vi "Get Format Test Settings.vi"(8 "Error In":errorcluster, 11 "Data Channel Ref In":T1 format="%.0x") -> (0 "Error Out":errorcluster, 2 "Data Channel Settings":T2, 3 "Data Channel Ref Out":T1 format="%.0x")   [LabVIEW 2018, in "Instrument Addon Scripting API Channels Unit Tests.lvclass"]
uses:
  Instrument Addon Scripting API Channels Unit Tests.lvclass
  <vilib>/NI Veristand/Custom Device API/Custom Device Item Ref.ctl
  APIs/Scripting API/TypeDefs/Array Format Settings.ctl
  APIs/Scripting API/TypeDefs/Array Element.ctl
  <vilib>/NI Veristand/Custom Device API/Get Item Property (String).vi
  <vilib>/NI Veristand/Custom Device API/Custom Device API.lvlib
  APIs/Scripting API/Instrument Addon Scripting API.lvlib
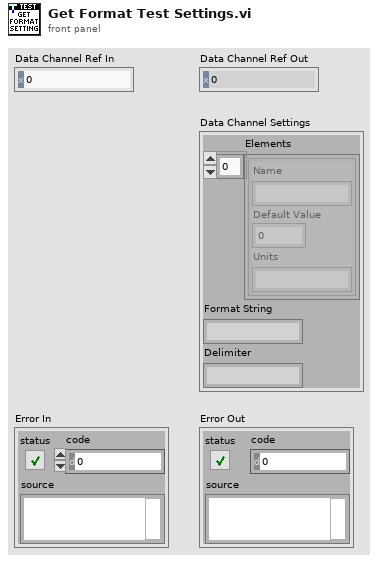
[diagram p1: front panel]
types:
  T1 = typedef "Custom Device API.lvlib/Custom Device Item Ref.ctl" = u64
  T2 = typedef "Instrument Addon Scripting API.lvlib/Array Format Settings.ctl" = cluster{"Elements":T3[], "Format String":string, "Delimiter":string}
  T3 = typedef "Instrument Addon Scripting API.lvlib/Array Element.ctl" = cluster{"Name":string, "Default Value":dbl, "Units":string}
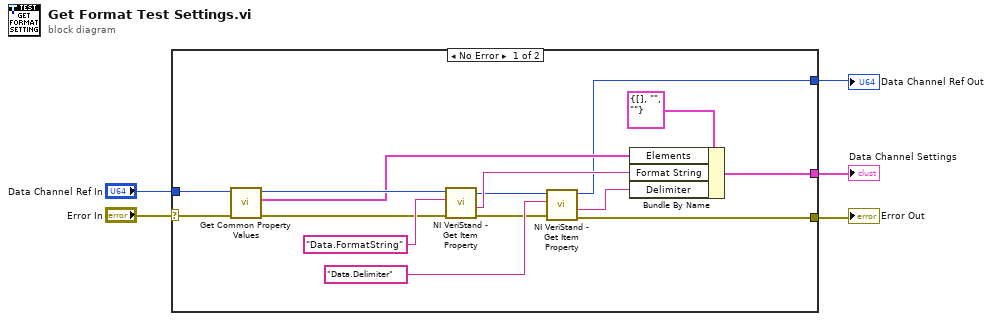
[diagram p0: block diagram]
diagram:
  n1 = case shown="No Error" "Error In" {
    selector: "Error In" -> [w6 w21]
    tunnel: [w20 _] -> w5
    tunnel: [w17 w21] -> w4
    tunnel: "Data Channel Ref In" -> [w11 w22]
    tunnel: [w7 w22] -> w1
    frame No Error {
      n2 = call "Get Common Property Values.vi"("Error In"=w6, "Data Channel  Ref in"=w11) -> ("error out"=w10:errorcluster, "Array Out"=w8:T3[], "Data Channel Ref Out"=w9:u64)  [unwired: 7 in]
      n3 = call-poly <vilib>:"NI VeriStand - Get Item Property.vi"("error in (no error)"=w10, "Property Name"="Data.FormatString", "Item Ref in"=w9) -> ("error out"=w13:errorcluster, "Value"=w19:string, "Item Ref out"=w14:T1)  [unwired: 5 in, 1 out]
      n4 = call-poly <vilib>:"NI VeriStand - Get Item Property.vi"("error in (no error)"=w13, "Property Name"="Data.Delimiter", "Item Ref in"=w14) -> ("error out"=w17:errorcluster, "Value"=w16:string, "Item Ref out"=w7:T1)  [unwired: 5 in, 1 out]
      n5 = Bundle By Name(cluster=T2 {"Elements"=[], "Format String"="", "Delimiter"=""} ("Settings"), "Elements"=w8, "Format String"=w19, "Delimiter"=w16) -> (w20:T2)
    }
    frame Error {
    }
  }
  "Data Channel Settings" <- w5
  "Error Out" <- w4
  "Data Channel Ref Out" <- w1
